vi "Initialize and Configure Cam.vi"(7 "Number of Buffers":u32=5, 8 "error in":errorcluster, 9 "Continuous?":T1, 10 "Camera Control Mode":T2, 11 "Camera name":string) -> (0 "error out":errorcluster, 3 "camera session out":T3)   [LabVIEW 2021, in "ImageStreamRendering.lvlib"]
uses:
  ImageStreamRendering.lvlib
  <vilib>/userdefined/High Color/IMAQdx.ctl
  <vilib>/vision/driver/IMAQdx.llb/IMAQdx Camera Control Mode.ctl
  <vilib>/vision/driver/IMAQdx.llb/IMAQdx Acquisition Mode.ctl
  <vilib>/vision/driver/NI_Vision_Acquisition_Software.lvlib
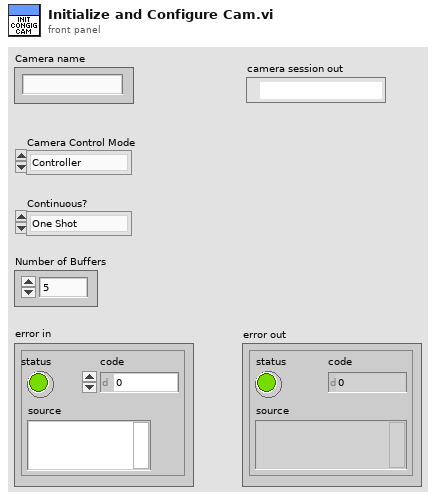
[diagram p1: front panel]
types:
  T1 = typedef "NI_Vision_Acquisition_Software.lvlib/IMAQdx Acquisition Mode.ctl" = enum32{"One Shot", "Continuous"}
  T2 = typedef "NI_Vision_Acquisition_Software.lvlib/IMAQdx Camera Control Mode.ctl" = enum32{"Controller", "Listener"}
  T3 = typedef "IMAQdx.ctl" = refnum<k21>
  T4 = typedef "IMAQ Image.ctl" = refnum<image>
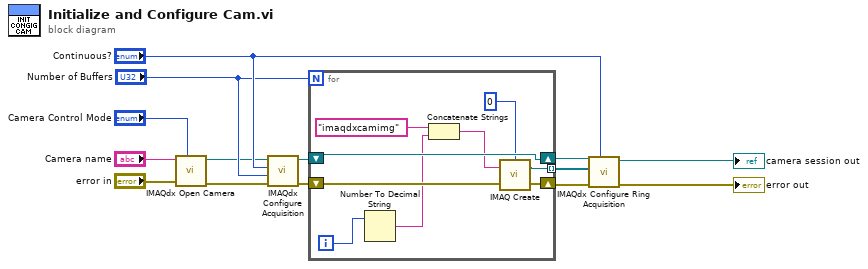
[diagram p0: block diagram]
diagram:
  n1 = call <vilib>:"IMAQdx Open Camera.vi"("Camera Control Mode"="Camera Control Mode", "error in"="error in", "Session In"="Camera name") -> ("error out"=w5:errorcluster, "Session Out"=w4:T3)  [unwired: 7 in]
  n2 = call <vilib>:"IMAQdx Configure Acquisition.vi"("error in"=w5, "Number of Buffers"="Number of Buffers", "Continuous?"="Continuous?", "Session In"=w4) -> ("error out"=w6:errorcluster, "Session Out"=w8:T3)  [unwired: 6 in]
  n3 = for {
    N: "Number of Buffers" -> [_]
    shift-right: [w21] -> w11
    shift-left: w6 -> [w22]
    tunnel: [w20] -> w10 mode=indexing
    shift-right: [w19] -> w9
    shift-left: w8 -> [w19]
    i -> [w16]
    n4 = Number To Decimal String(number=w16) -> (decimal integer string=w15:string)  [unwired: 1 in]
    n5 = Concatenate Strings("imaqdxcamimg" ("Image Name"), w15) -> (w17:string)
    n6 = call "IMAQ Create"("Border Size"=0, "Image Name"=w17, "error in (no error)"=w22) -> ("New Image"=w20:T4, "error out"=w21:errorcluster)  [unwired: 2 in]
  }
  n7 = call <vilib>:"IMAQdx Configure Ring Acquisition.vi"("Mode"="Continuous?", "error in"=w11, "Images"=w10, "Session In"=w9) -> ("error out"=→"error out":errorcluster, "Session Out"=→"camera session out":T3)  [unwired: 5 in, 1 out]
